vi "Set BG Color.vi"(8 "error in (no error)":errorcluster, 10 "BG":u32(colorbox), 11 "SubClone in":refnum<class "SubClone.lvclass">) -> (0 "error out":errorcluster, 3 "SubClone out":refnum<class "SubClone.lvclass">)   [LabVIEW 2020, in "SubPanels.lvlib" / "SubClone.lvclass"]
uses:
  SubClone.lvclass
  SubClone.lvclass/SubClone.ctl
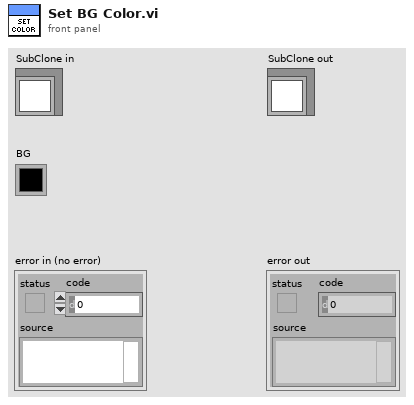
[diagram p1: front panel]
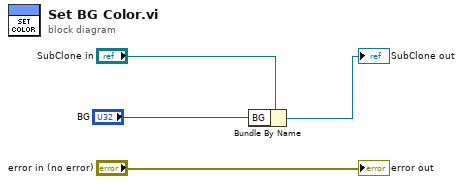
[diagram p0: block diagram]
diagram:
  n1 = Bundle By Name(cluster="SubClone in", "BG"="BG") -> (→"SubClone out":refnum<class "SubClone.lvclass">)
  "error out" <- "error in (no error)"
